vi "Post Tweet with Pic.vi"(8 "error in":errorcluster, 10 "Picture File (PNG, JPG, GIF)":path, 11 "Tweet":string) -> (0 "error out":errorcluster)   [LabVIEW 2019]
doc: "This example posts a tweet and picture from a file. Permitted file types are .jpg, .jpeg, .gif, and .bmp. Animated gifs are not allowed."
uses:
  <vilib>/LVH/i3 Twitter/SubVIs/Twitter Open - Embedded.vi
  <vilib>/LVH/i3 Twitter/Tweets with Media/Post Media Tweet - From File.vi
  <vilib>/LVH/i3 Twitter/i3-twitter.lvlib
panel:
  in  "Access Secret":string
  in  "Access Token":string
  in  "Consumer Secret":string
  in  "Consumer Key":string
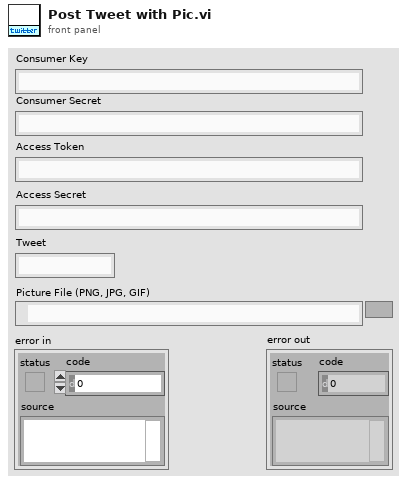
[diagram p1: front panel]
types:
  T1 = typedef "i3-twitter.lvlib/Twitter Handle.ctl" = cluster{"OAuth Credentials":T2, "since ID":string, "max ID":string, "Screen Name":string}
  T2 = typedef "i3-oauth.lvlib/OAuth Handle.ctl" = cluster{"Signature Method":T3, "Version":string, "Client":T4, "Access":T4}
  T3 = typedef "i3-oauth.lvlib/Signature Method.ctl" = enum16{"HMAC-MD5", "HMAC-SHA1", "HMAC-SHA224", "HMAC-SHA256", "HMAC-SHA384", "HMAC-SHA512"}
  T4 = typedef "i3-oauth.lvlib/Credentials.ctl" = cluster{"Token":string, "Secret":string}
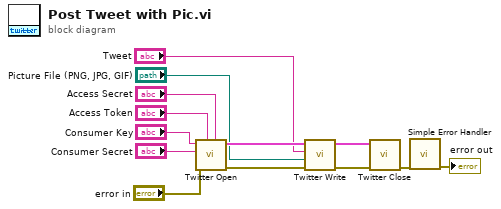
[diagram p0: block diagram]
diagram:
  n1 = call-poly <vilib>:"Twitter Open.vi"("Access Secret"="Access Secret", "Access Token"="Access Token", "error in"="error in", "Consumer Secret"="Consumer Secret", "Consumer Key"="Consumer Key") -> ("error out"=w13:errorcluster, "Twitter Handle Out"=w11:T1)  [unwired: 5 in]
  n2 = call-poly <vilib>:"Twitter Write.vi"("error in"=w13, "Picture File (PNG, JPG, GIF)"="Picture File (PNG, JPG, GIF)", "Tweet"="Tweet", "Twitter Handle In"=w11) -> ("error out"=w12:errorcluster, "Twitter Handle Out"=w10:T1)  [unwired: 6 in]
  n3 = call <vilib>:"Twitter Close.vi"("error in"=w12, "Twitter Handle In"=w10) -> ("error out"=w7:errorcluster)  [unwired: 9 in]
  n4 = call <vilib>:"Simple Error Handler.vi"("error in (no error)"=w7) -> ("error out"=→"error out":errorcluster)  [unwired: 4 in, 4 out]
